vi "Auton Builder.vi"() -> ()   [LabVIEW 2019]
uses:
  Typedef/Robot Settings.ctl
  Typedef/Data Point.ctl
  Typedef/Robot Starting Position.ctl
  <vilib>/Rock Robotics/WPI/ThirdParty/WPILib Extensions/Trajectory/Typedef/Differential Drive Constraints.ctl
  <vilib>/Rock Robotics/WPI/ThirdParty/WPILib Extensions/Trajectory/Typedef/Differential Drive Constants.ctl
  Typedef/Landmark Definition.ctl
  Typedef/Sequence Command.ctl
  Typedef/Plate Arrangement.ctl
  <vilib>/Utility/miscctls.llb/LVRowAndColumnTypeDef.ctl
  <vilib>/Rock Robotics/WPI/ThirdParty/WPILib Extensions/Geometry/Typedef/Pose2d.ctl
  <vilib>/Rock Robotics/WPI/ThirdParty/WPILib Extensions/Geometry/Typedef/Translation2d.ctl
  <vilib>/Rock Robotics/WPI/ThirdParty/WPILib Extensions/Geometry/Typedef/Rotation2d.ctl
panel:
  in  "Start Position Names":T1=enum."Center"
  in  "Stop?":bool
  in  "Tab Control":enum32{"Builder", "Raw Sequence", "Settings"}(tab)
  in  "Landmarks":u16(ring) items=["Left Wall Start"]
  in  "Insert Landmark":bool
  in  "Alliance":bool
  out "Field Half":cluster{dbl[], dbl[]}[](graph)=[{[48.5, 82.0, 82.0, 48.5, 48.5], [176.25, 176.25, 147.75, 147.75, 176.25]}, {[68.0], [162.0]}, {[68.0], [162.0]}, {[81.13940299900052], [156.48469503745656]}, {[54.86059700099948], [167.51530496254344]}]
  in  "Start Position":T1=enum."Center"
  in  "Reverse Path":bool
  in  "Data Points":T2[](array[typedef])=[{"X"=68.0, "Y"=162.0, "Theta"=0.0, "Speed %"=0.0, "Disabled?"=FALSE}]
  in  "Open":bool
  in  "Save":bool
  in  "Reset":bool
  in  "Send to Robot":bool
  in  "Simulate":bool
  in  "Name":string
  in  "Cancel":bool
  out "Total Time Seconds":dbl
  in  "Lardmark List":T3[](array[typedef])=[{"X Red"=140.0, "Y Red"=305.0, "Theta Red"=0.0, "X Blue"=140.0, "Y Blue"=305.0, "Theta Blue"=0.0, "Name"="Left Wall Start"}]
  out "Location Names":string[](array[string])=["Top Center", "Center", "Bottom Center", "Top Railing"]
  in  "Locations":cluster{"X":dbl, "Y":dbl}[](array[cluster])=[{"X"=120.0, "Y"=266.0}, {"X"=120.0, "Y"=228.0}, {"X"=120.0, "Y"=187.0}, {"X"=120.0, "Y"=297.0}, {"X"=140.0, "Y"=305.0}]
  in  "Path Folder":path=path "C:/Users/RoboChargers/Documents/LabVIEW Data/Deep-Space-2019/Auton/Paths"
  in  "Robot Settings":T4={"Width"=0.6, "Length"=0.7, "Center of Rotation"=0.2} caption="Robot Settings w/ Bumpers"
  in  "Constants":T5={"ks"=0.162, "kv"=2.71, "ka"=0.468, "trackwidth"=0.67163}
  in  "Constraints":T6={"maxVoltage"=9.0, "maxVelocity"=3.0, "maxAccel"=1.5}
  # "LEFT"
  # "+Y"
  # "FAR"
  # "+X"
  # "NEAR"
  # "RIGHT"
  # "Counter Clockwise Positive\n+X = 0 degrees"
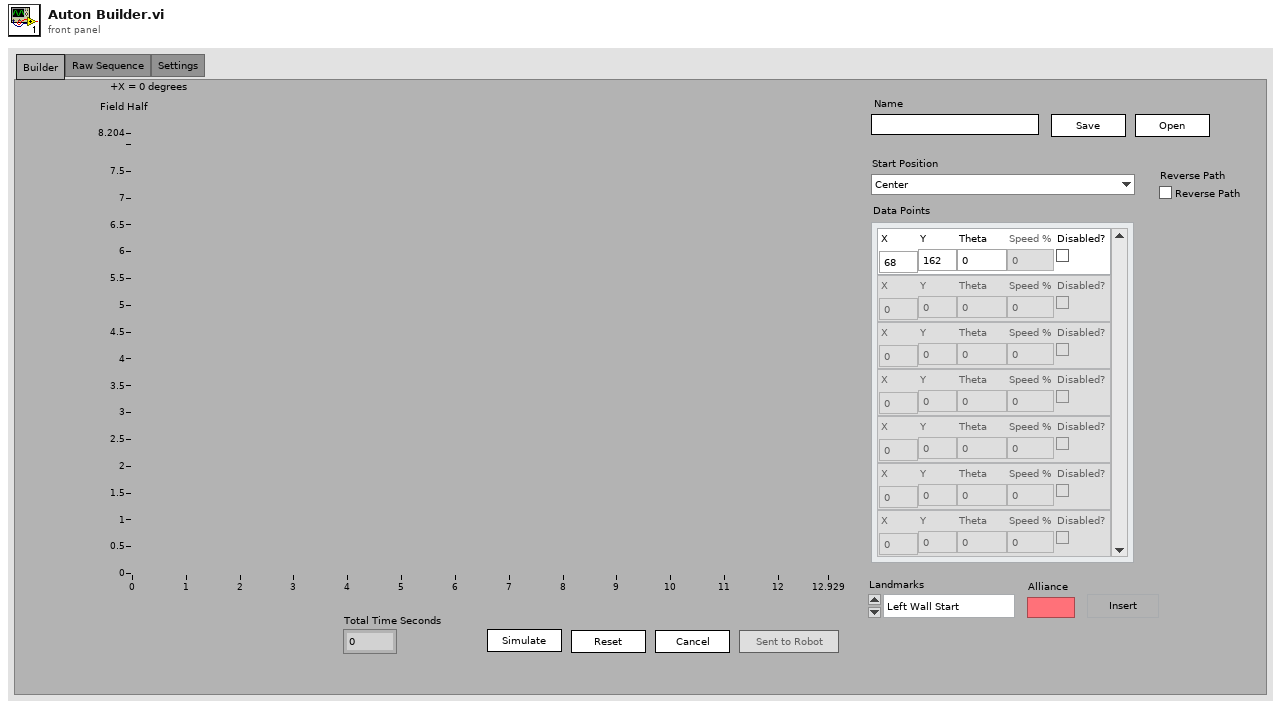
[diagram p1: front panel]
types:
  T1 = typedef "Robot Starting Position.ctl" = enum16{"Left Center", "Center", "Bottom Center", "Left Trench", "Left Wall"}
  T2 = typedef "Data Point.ctl" = cluster{"X":dbl, "Y":dbl, "Theta":dbl, "Speed %":dbl, "Disabled?":bool}
  T3 = typedef "Landmark Definition.ctl" = cluster{"X Red":dbl, "Y Red":dbl, "Theta Red":dbl, "X Blue":dbl, "Y Blue":dbl, "Theta Blue":dbl, "Name":string}
  T4 = typedef "Robot Settings.ctl" = cluster{"Width":dbl, "Length":dbl, "Center of Rotation":dbl}
  T5 = typedef "Differential Drive Constants.ctl" = cluster{"ks":dbl, "kv":dbl, "ka":dbl, "trackwidth":dbl}
  T6 = typedef "Differential Drive Constraints.ctl" = cluster{"maxVoltage":dbl, "maxVelocity":dbl, "maxAccel":dbl}
  T7 = typedef "Sequence Command.ctl" = cluster{"Sequence Name":string, "Plate Arrangement":T8, "Command Name":string, "Data":variant, "Sequence Number":u32}
  T8 = typedef "Plate Arrangement.ctl" = cluster{"LR*":bool, "LL*":bool, "RL*":bool, "RR*":bool}
  T9 = typedef "LVRowAndColumnTypeDef.ctl" = cluster{"Row":i32, "Column":i32}
  T10 = cluster{"Field Half":cluster{dbl[], dbl[]}[], "Current Command":T7, "Robot Position":cluster{"x":dbl, "y":dbl}, "Theta":dbl, "y position":dbl, "Active Cell":T9, "Robot Index":i32, "Sequence OK?":bool, "Start Position":cluster{"x":dbl, "y":dbl}, "Field Selection":string, "Simulation Index":i32, "Sim Robot Index":i32, "Active Path":path, "Load Index":i32, "Graph Index":i32, "Data Points Index":i32, "Data Points":T2[], "Path Index":i32, "Path L Index":i32, "Path R Index":i32}
  T11 = typedef "Pose2d.ctl" = cluster{"Translation2d":T12, "Rotation2d":T13}
  T12 = typedef "Translation2d.ctl" = cluster{"x":dbl, "y":dbl}
  T13 = typedef "Rotation2d.ctl" = cluster{"Theta":dbl}
  T14 = typedef "Trajectory State.ctl" = cluster{"t":dbl, "velocity":dbl, "acceleration":dbl, "pose":T11, "curvature":dbl}
  T15 = typedef "LVPoint32TypeDef.ctl" = cluster{"Horizontal":i32, "Vertical":i32}
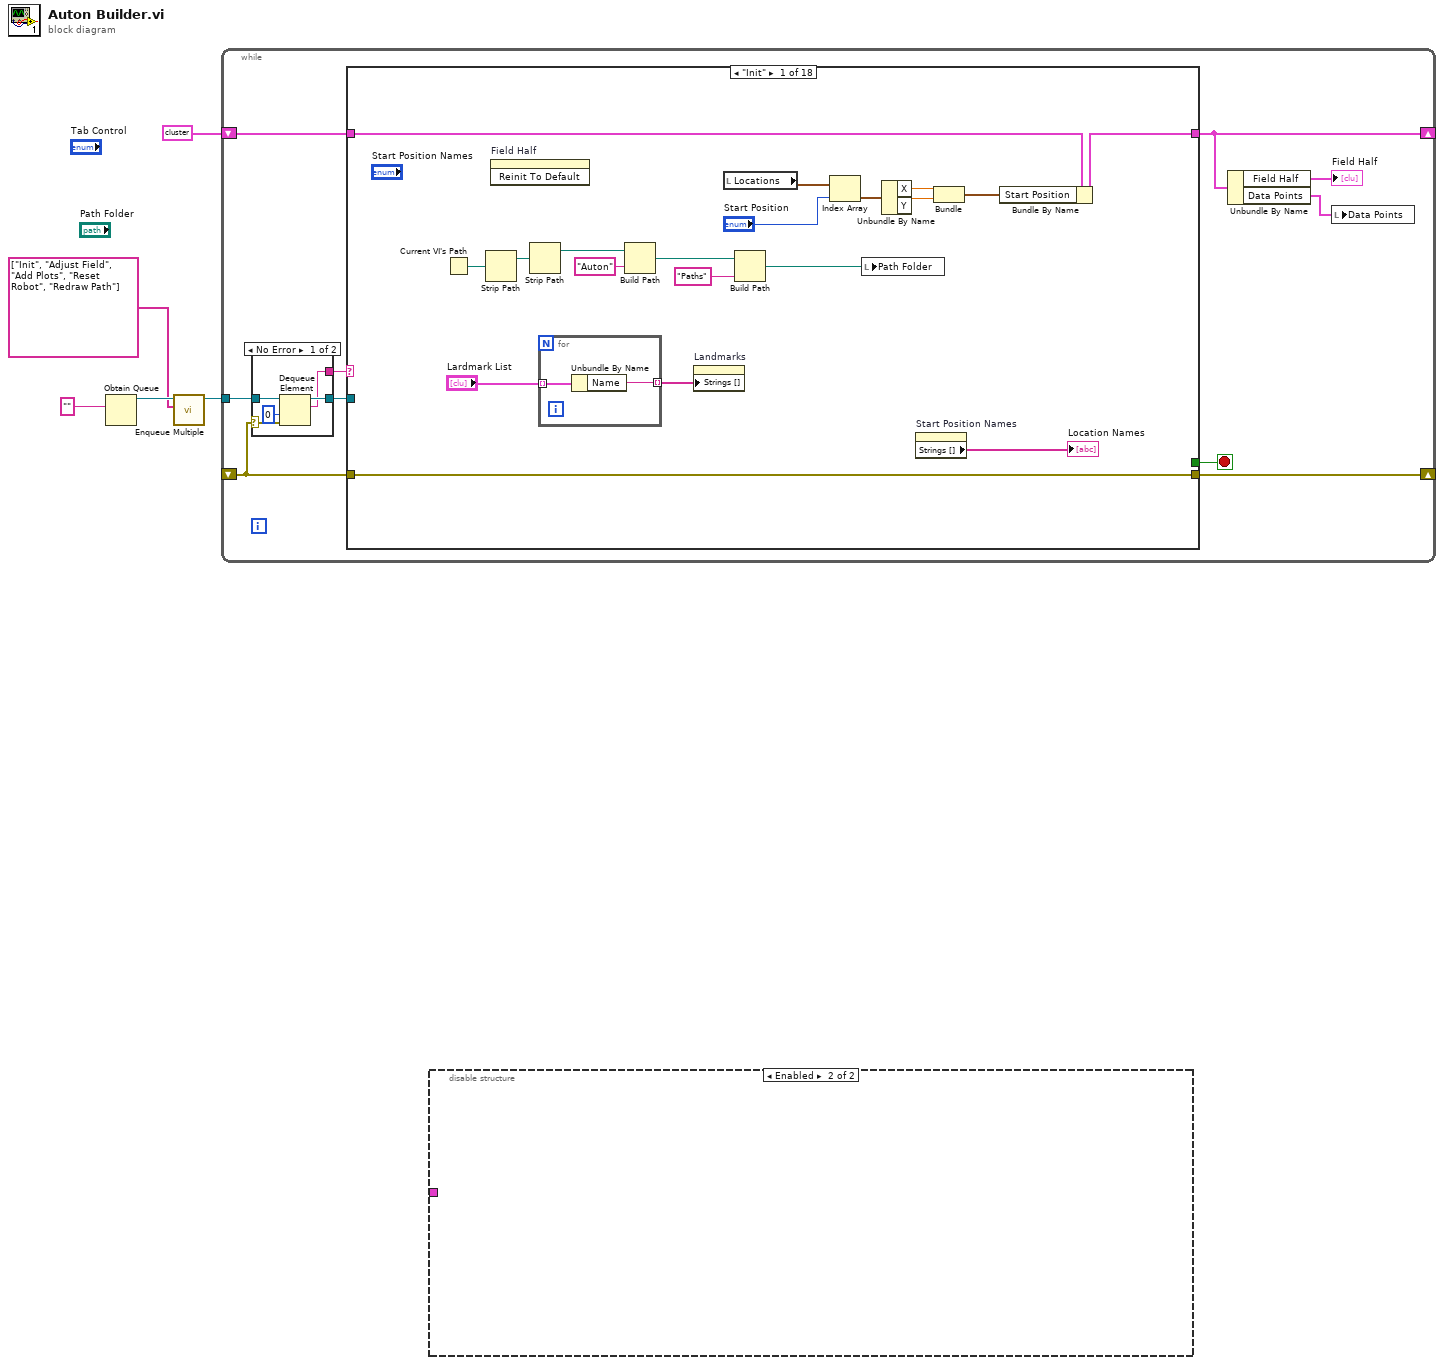
[diagram p0: block diagram]
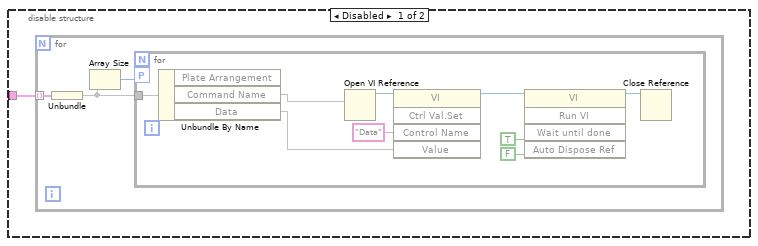
[diagram p2: hidden frame]
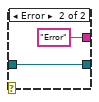
[diagram p3: hidden frame]
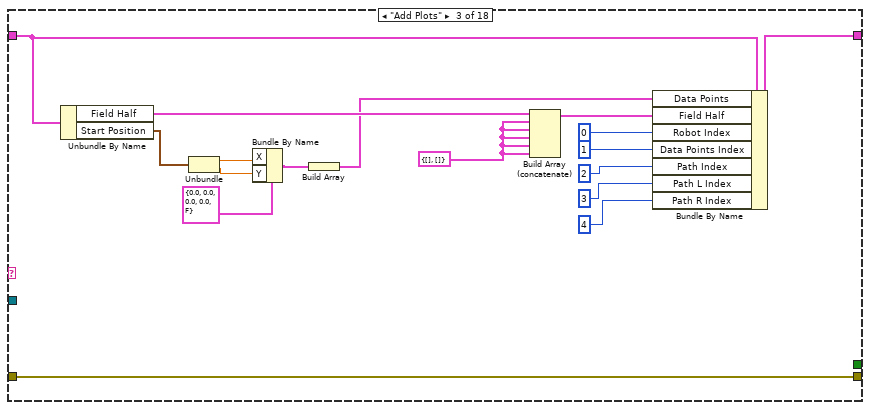
[diagram p5: hidden frame]
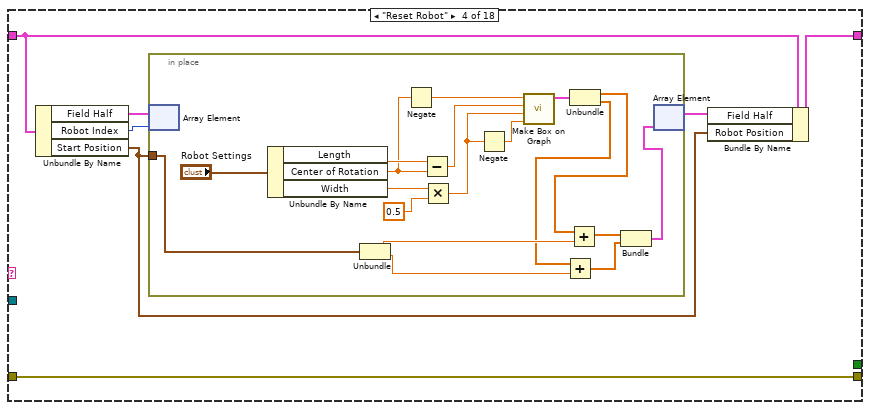
[diagram p6: hidden frame]
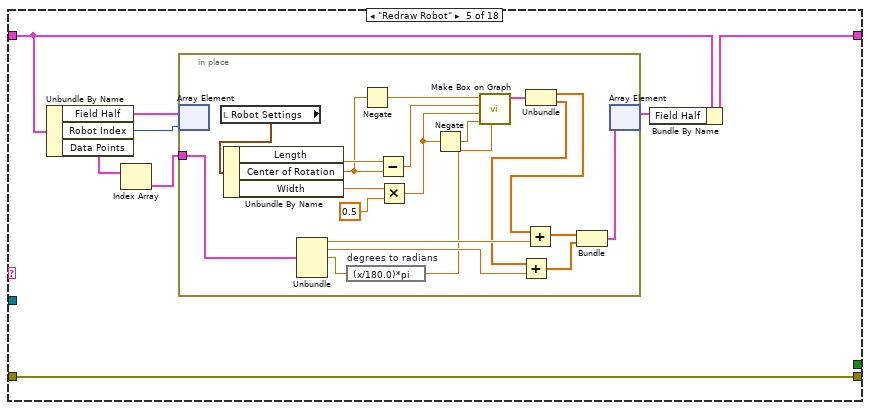
[diagram p7: hidden frame]
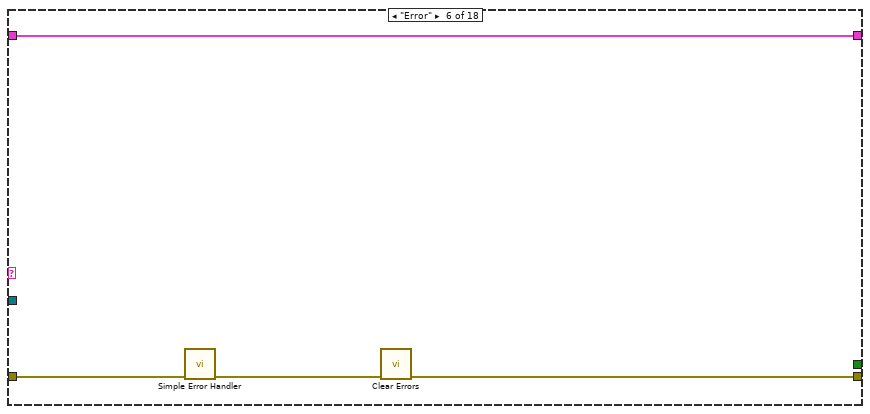
[diagram p8: hidden frame]
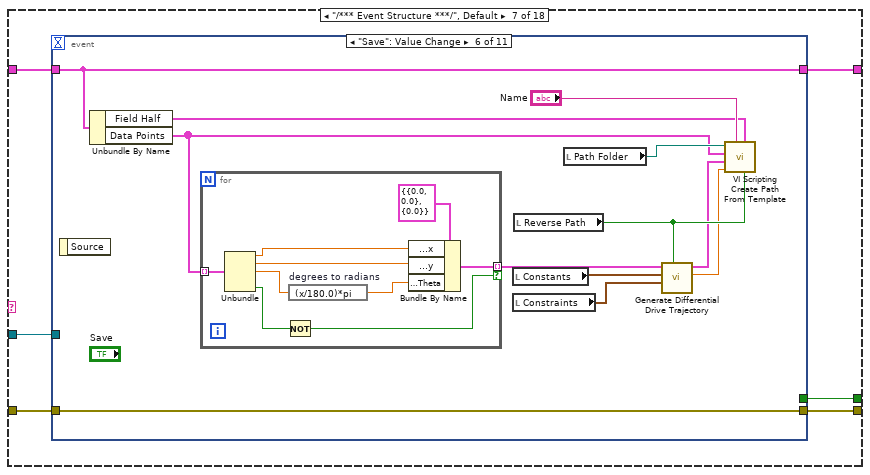
[diagram p9: hidden frame]
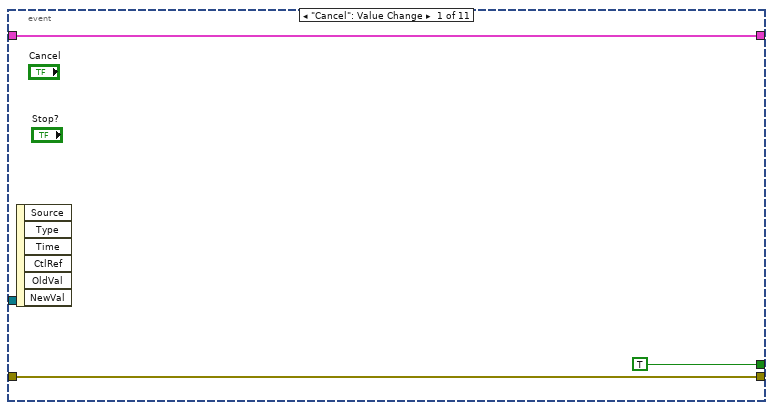
[diagram p10: hidden frame]
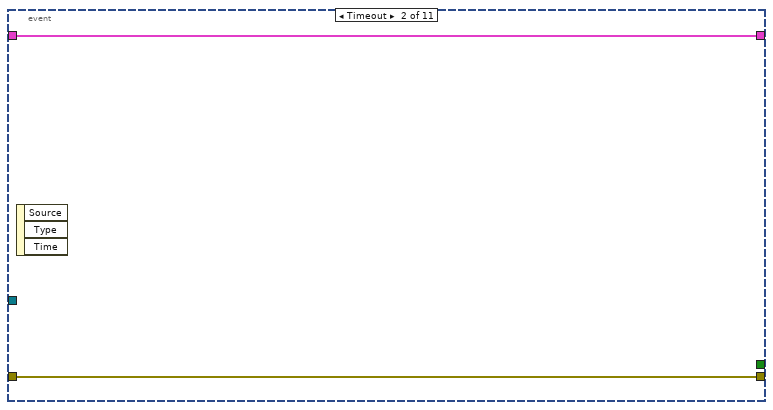
[diagram p11: hidden frame]
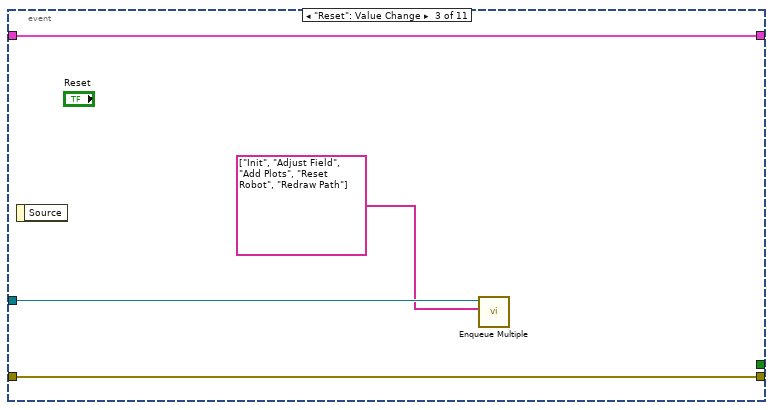
[diagram p12: hidden frame]
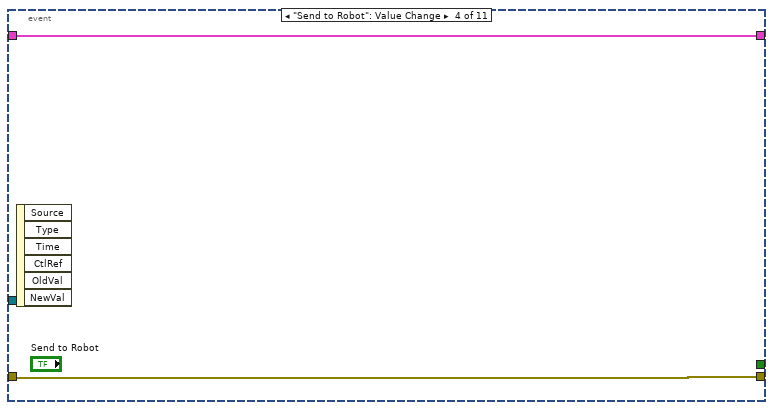
[diagram p13: hidden frame]
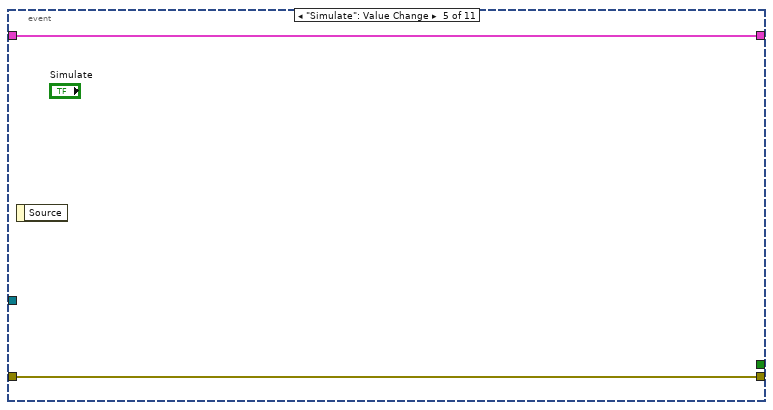
[diagram p14: hidden frame]
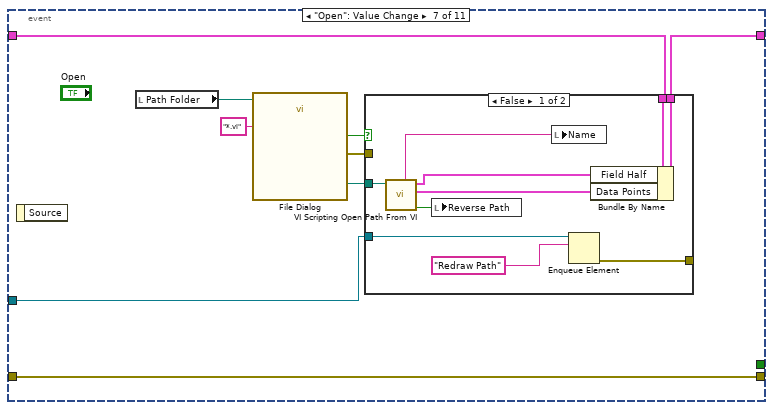
[diagram p15: hidden frame]
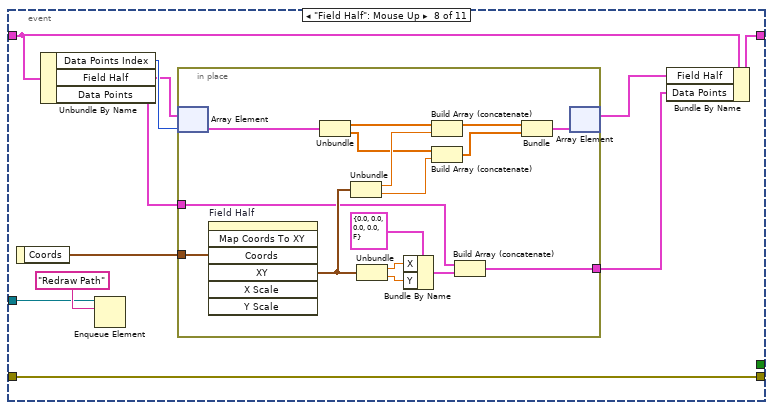
[diagram p17: hidden frame]
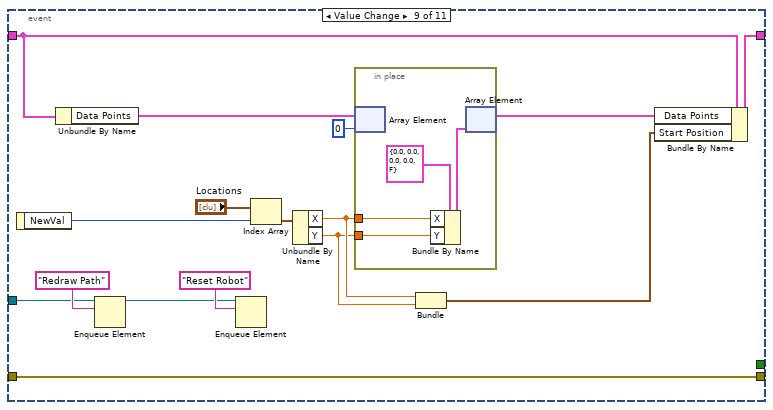
[diagram p18: hidden frame]
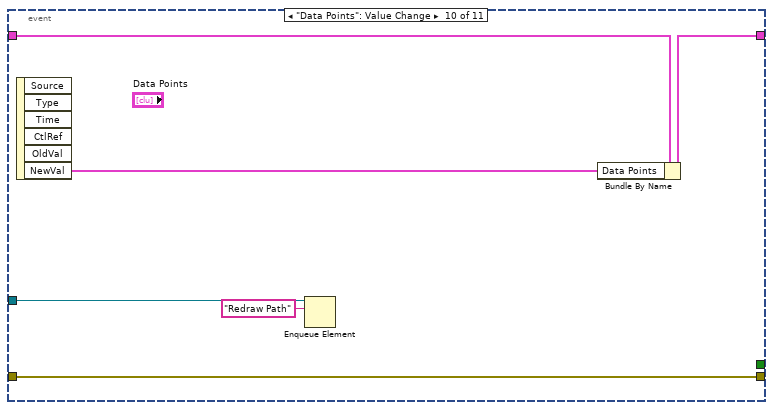
[diagram p19: hidden frame]
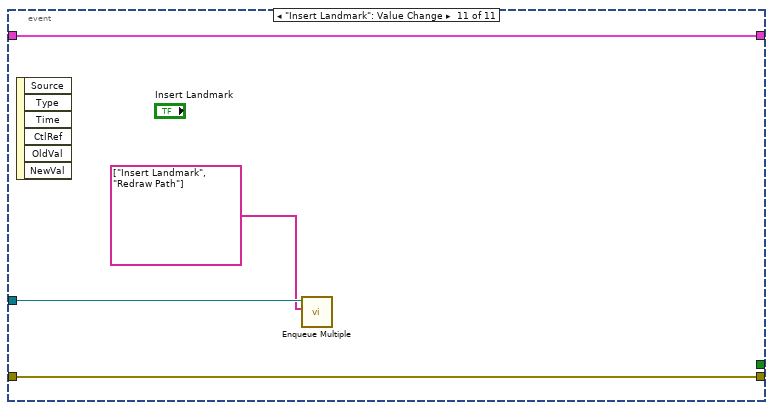
[diagram p20: hidden frame]
diagram:
  n1 = Obtain Queue(element data type="") -> (queue out=w4:refnum<queue>)  [unwired: 4 in, 2 out]
  n2 = call "Enqueue Multiple.vi"("Array"=string[] ["Init", "Adjust Field", "Add Plots", "Reset Robot", "Redraw Path"], "Queue in"=w4) -> ("Queue out"=w3:refnum<queue>)  [unwired: 8 in, 1 out]
  n3 = while {
    shift-right: [w9] -> _
    shift-left: T10 {"Field Half"=[], "Current Command"={"Sequence Name"="", "Plate Arrangement"={"LR*"=FALSE, "LL*"=FALSE, "RL*"=FALSE, "RR*"=FALSE}, "Command Name"="", "Data"=variant, "Sequence Number"=0}, "Robot Position"={"x"=0.0, "y"=0.0}, "Theta"=0.0, "y position"=0.0, "Active Cell"={"Row"=0, "Column"=0}, "Robot Index"=0, "Sequence OK?"=FALSE, "Start Position"={"x"=0.0, "y"=0.0}, "Field Selection"="", "Simulation Index"=0, "Sim Robot Index"=0, "Active Path"=path "", "Load Index"=0, "Graph Index"=0, "Data Points Index"=0, "Data Points"=[], "Path Index"=0, "Path L Index"=0, "Path R Index"=0} ("output cluster") -> [w15]
    shift-right: [w11] -> _
    shift-left: _ -> [w10]
    tunnel: w3 -> [w14]
    stop <- w7 stop-if-true
    n4 = case shown="No Error" w10 {
      selector: w10 -> [w18 _]
      tunnel: w14 -> [w20 w22]
      tunnel: [w19 w22] -> w13
      tunnel: [w17 "Error"] -> w12
      frame No Error {
        n5 = Dequeue Element(queue=w20, timeout in ms (-1)=0, error in (no error)=w18) -> (queue out=w19:refnum<queue>, element=w17:string)  [unwired: 2 out]
      }
      frame Error {
      }
    }
    n6 = case shown="\"Init\"" w12 {
      tunnel: [_ _ _ _ _ _ w125 _ _ _ _ _ _ _ _ _ _ _] -> w7
      tunnel: w15 -> [w41 w44 w60 w68 w94 w119 w124 w239 w251 w266 w278 w294 w336 w386 w401 w406 w408 w410]
      tunnel: [w40 w44 w62 w69 w95 w119 w123 w238 w244 w262 w277 w292 w334 w385 w401 w404 w408 w410] -> w9
      tunnel: w13 -> [_ _ _ _ _ _ w122 _ _ _ _ w285 w327 _ _ _ _ _]
      tunnel: [w39 w45 w58 w67 w93 w118 w120 w240 w242 w260 w279 w295 w337 w387 w400 w405 w407 w409] -> w11
      tunnel: w10 -> [w39 w45 w58 w67 w93 w117 w121 w240 w242 w260 w279 w295 w337 w387 w400 w405 w407 w409]
      frame "Init" {
        n7 = Current VI's Path() -> (path=w38:path)
        n8 = Strip Path(path=w38) -> (stripped path=w37:path)  [unwired: 1 out]
        n9 = invoke on="Field Half" class="XYGraph (strict)" method="Reinit To Default"() -> ()  [unwired: 3 in, 3 out]
        n10 = Strip Path(path=w37) -> (stripped path=w36:path)  [unwired: 1 out]
        n11 = for {
          tunnel: [w42] -> w23 mode=indexing
          tunnel: "Lardmark List" -> [w43] mode=indexing
          n12 = Unbundle By Name(w43) -> ("Name"=w42:string)
        }
        n13 = Build Path(base path=w36, name or relative path="Auton") -> (appended path=w34:path)
        n14 = property on="Landmarks" class="Ring (strict)"("Strings []"=w23) -> ()  [unwired: 2 in, 2 out]
        n15 = local read "Locations"() -> (w26:cluster{"X":dbl, "Y":dbl}[])
        n16 = Build Path(base path=w34, name or relative path="Paths") -> (appended path=w32:path)
        n17 = Index Array(array=w26, index="Start Position") -> (element=w30:cluster{"X":dbl, "Y":dbl})
        n18 = local write "Path Folder"(w32) -> ()
        n19 = Unbundle By Name(w30) -> ("X"=w29:dbl, "Y"=w28:dbl)
        n20 = property on="Start Position Names" class="Enum (strict)"() -> ("Strings []"=→"Location Names":string[])  [unwired: 2 in, 2 out]
        n21 = Bundle("X"=w29, "Y"=w28) -> (w27:cluster{"X":dbl, "Y":dbl})  [unwired: 1 in]
        n22 = Bundle By Name(cluster=w41, "Start Position"=w27) -> (w40:T10)
      }
      frame "Adjust Field" {
      }
      frame "Add Plots" {
        w51 = cluster{dbl[], dbl[]} {[], []} ("element")
        n23 = Unbundle By Name(w60) -> ("Field Half"=w59:cluster{dbl[], dbl[]}[], "Start Position"=w52:cluster{"x":dbl, "y":dbl})
        n24 = Unbundle(w52) -> ("x"=w49:dbl, "y"=w48:dbl)
        n25 = Bundle By Name(cluster=T2 {"X"=0.0, "Y"=0.0, "Theta"=0.0, "Speed %"=0.0, "Disabled?"=FALSE} ("Cluster"), "X"=w49, "Y"=w48) -> (w47:T2)
        n26 = Build Array(w47) -> (w46:T2[])
        n27 = Build Array (concatenate)(w59, w51, w51, w51, w51, w51) -> (w61:cluster{dbl[], dbl[]}[])
        n28 = Bundle By Name(cluster=w60, "Data Points"=w46, "Field Half"=w61, "Robot Index"=0, "Data Points Index"=1 ("Spline Index"), "Path Index"=2 ("Spline Index"), "Path L Index"=3 ("Spline Index"), "Path R Index"=4 ("Spline Index")) -> (w62:T10)
      }
      frame "Reset Robot" {
        n29 = Unbundle By Name(w68) -> ("Field Half"=w66:cluster{dbl[], dbl[]}[], "Robot Index"=w65:i32, "Start Position"=w63:cluster{"x":dbl, "y":dbl})
        n30 = in-place {
          in-place-border: w63 -> [w87]
          n31 = in-place-array #1(w66, w65) -> ()  [unwired: 1 out]
          n32 = Unbundle By Name("Robot Settings") -> ("Length"=w77:dbl, "Center of Rotation"=w76:dbl, "Width"=w81:dbl)
          n33 = Unbundle(w87) -> ("x"=w86:dbl, "y"=w85:dbl)
          n34 = Negate(x=w76) -> (-x=w78:dbl)
          n35 = Subtract(x=w77, y=w76) -> (x-y=w75:dbl)
          n36 = Multiply(x=w81, y=0.5 ("x")) -> (x*y=w80:dbl)
          n37 = Negate(x=w80) -> (-x=w79:dbl)
          n38 = call "Make Box on Graph.vi"("Y2"=w79, "Y1"=w80, "X2"=w75, "X1"=w78) -> ("Output Graph"=w73:cluster{dbl[], dbl[]})  [unwired: 7 in]
          n39 = Unbundle(w73) -> (w72:dbl[], w71:dbl[])
          n40 = Add(x=w71, y=w85) -> (x+y=w84:dbl[])
          n41 = Add(x=w72, y=w86) -> (x+y=w83:dbl[])
          n42 = Bundle(w83, w84) -> (w70:cluster{dbl[], dbl[]})  [unwired: 1 in]
          n43 = in-place-array #1(w70) -> (w64:cluster{dbl[], dbl[]}[])  [unwired: 1 out]
        }
        n44 = Bundle By Name(cluster=w68, "Field Half"=w64, "Robot Position"=w63) -> (w69:T10)
      }
      frame "Redraw Robot" {
        n45 = Unbundle By Name(w94) -> ("Field Half"=w92:cluster{dbl[], dbl[]}[], "Robot Index"=w91:i32, "Data Points"=w90:T2[])
        n46 = Index Array(array=w90) -> (element=w89:T2)  [unwired: 1 in]
        n47 = in-place {
          in-place-border: w89 -> [w115]
          n48 = in-place-array #2(w92, w91) -> ()  [unwired: 1 out]
          n49 = local read "Robot Settings"() -> (w99:T4)
          n50 = Unbundle By Name(w99) -> ("Length"=w106:dbl, "Center of Rotation"=w105:dbl, "Width"=w110:dbl)
          n51 = Unbundle(w115) -> ("X"=w114:dbl, "Y"=w113:dbl, "Theta"=w97:dbl)  [unwired: 2 out]
          n52 = expression code="(x/180.0)*pi" "degrees to radians"(w97) -> (w96:dbl)
          n53 = Negate(x=w105) -> (-x=w107:dbl)
          n54 = Subtract(x=w106, y=w105) -> (x-y=w104:dbl)
          n55 = Multiply(x=w110, y=0.5 ("x")) -> (x*y=w109:dbl)
          n56 = Negate(x=w109) -> (-x=w108:dbl)
          n57 = call "Make Box on Graph.vi"("Theta"=w96, "Y2"=w108, "Y1"=w109, "X2"=w104, "X1"=w107) -> ("Output Graph"=w102:cluster{dbl[], dbl[]})  [unwired: 6 in]
          n58 = Unbundle(w102) -> (w101:dbl[], w100:dbl[])
          n59 = Add(x=w100, y=w113) -> (x+y=w112:dbl[])
          n60 = Add(x=w101, y=w114) -> (x+y=w111:dbl[])
          n61 = Bundle(w111, w112) -> (w98:cluster{dbl[], dbl[]})  [unwired: 1 in]
          n62 = in-place-array #2(w98) -> (w88:cluster{dbl[], dbl[]}[])  [unwired: 1 out]
        }
        n63 = Bundle By Name(cluster=w94, "Field Half"=w88) -> (w95:T10)
      }
      frame "Error" {
        n64 = call <vilib>:"Simple Error Handler.vi"("error in (no error)"=w117) -> ("error out"=w116:errorcluster)  [unwired: 4 in, 4 out]
        n65 = call <vilib>:"Clear Errors.vi"("error in (no error)"=w116) -> ("error out"=w118:errorcluster)  [unwired: 5 in, 1 out]
      }
      frame "/*** Event Structure ***/", Default {
        n66 = event shown="[5] \"Save\": Value Change" {
          selector: _ -> [_ _ _ _ _ _ _ _ _ _ _]
          dyn-events: _ -> [_ _ _ _ _ _ _ _ _ _ _]
          timeout: _ -> [_ _ _ _ _ _ _ _ _ _ _]
          tunnel: [TRUE _ _ _ _ _ _ _ _ _ _] -> w125
          tunnel: w124 -> [w127 w130 w134 w136 w138 w150 w162 w186 w221 w231 w233]
          tunnel: [w127 w130 w134 w136 w138 w150 w161 w184 w220 w230 w233] -> w123
          tunnel: w122 -> [_ _ w133 _ _ _ w160 w180 w218 w228 w235]
          tunnel: w121 -> [w126 w129 w132 w135 w137 w148 w168 w190 w222 w232 w236]
          tunnel: [w126 w129 w132 w135 w137 w148 w168 w190 w222 w232 w236] -> w120
          event "Cancel": Value Change {
            n67 = event-data() -> ()  [unwired: 1 in, 6 out]
          }
          event Timeout {
            n68 = event-data() -> ()  [unwired: 1 in, 3 out]
          }
          event "Reset": Value Change {
            n69 = event-data() -> ()  [unwired: 1 in, 1 out]
            n70 = call "Enqueue Multiple.vi"("Array"=string[] ["Init", "Adjust Field", "Add Plots", "Reset Robot", "Redraw Path"], "Queue in"=w133) -> ()  [unwired: 8 in, 2 out]
          }
          event "Send to Robot": Value Change {
            n71 = event-data() -> ()  [unwired: 1 in, 6 out]
          }
          event "Simulate": Value Change {
            n72 = event-data() -> ()  [unwired: 1 in, 1 out]
          }
          event "Save": Value Change {
            n73 = event-data() -> ()  [unwired: 1 in, 1 out]
            n74 = Unbundle By Name(w150) -> ("Field Half"=w146:cluster{dbl[], dbl[]}[], "Data Points"=w142:T2[])
            n75 = for {
              tunnel: w142 -> [w159] mode=indexing
              tunnel: [w157] -> w145 mode=indexing if=w155
              n76 = Unbundle(w159) -> ("X"=w151:dbl, "Y"=w152:dbl, "Theta"=w153:dbl, "Disabled?"=w156:bool)  [unwired: 1 out]
              n77 = Not(x=w156) -> (.not. x?=w155:bool)
              n78 = expression code="(x/180.0)*pi" "degrees to radians"(w153) -> (w154:dbl)
              n79 = Bundle By Name(cluster=T11 {"Translation2d"={"x"=0.0, "y"=0.0}, "Rotation2d"={"Theta"=0.0}} ("pose"), "Translation2d.x"=w151, "Translation2d.y"=w152, "Rotation2d.Theta"=w154) -> (w157:T11)
            }
            n80 = local read "Constants"() -> (w143:T5)
            n81 = local read "Constraints"() -> (w144:T6)
            n82 = local read "Reverse Path"() -> (w141:bool)
            n83 = local read "Path Folder"() -> (w147:path)
            n84 = call <vilib>:"Generate Differential Drive Trajectory.vi"("Reverse?"=w141, "Constraints"=w144, "Constants"=w143, "Waypoints"=w145) -> ("Total Time Seconds"=w139:dbl, "states"=w140:T14[])  [unwired: 5 in, 1 out]
            n85 = call "VI Scripting Create Path From Template.vi"("Reverse Path?"=w141, "Graph"=w146, "Name"="Name", "Total Time (s)"=w139, "Trajectory"=w140, "Data Points"=w142, "base path"=w147) -> ()  [unwired: 5 in]
          }
          event "Open": Value Change {
            n86 = event-data() -> ()  [unwired: 1 in, 1 out]
            n87 = local read "Path Folder"() -> (w166:path)
            n88 = call "File Dialog"("start path"=w166, "pattern (all files)"="*.vi") -> ("selected path"=w167:path, "cancelled"=w165:bool, "error out"=w164:errorcluster)  [unwired: 10 in, 1 out]
            n89 = case shown="False" w165 {
              tunnel: w167 -> [w178 _]
              tunnel: w162 -> [w177 w179]
              tunnel: [w175 w179] -> w161
              tunnel: w160 -> [w172 _]
              tunnel: w164 -> [_ _]
              tunnel: [w169 _] -> _
              frame False {
                n90 = call "VI Scripting Open Path From VI.vi"("Path"=w178) -> ("Reverse Path?"=w176:bool, "Data Points"=w173:T2[], "Graph"=w174:cluster{dbl[], dbl[]}[], "Name"=w170:string)  [unwired: 6 in, 1 out]
                n91 = local write "Reverse Path"(w176) -> ()
                n92 = local write "Name"(w170) -> ()
                n93 = Enqueue Element(queue=w172, element="Redraw Path") -> (error out=w169:errorcluster)  [unwired: 2 in, 2 out]
                n94 = Bundle By Name(cluster=w177, "Field Half"=w174, "Data Points"=w173) -> (w175:T10)
              }
              frame True {
              }
            }
          }
          event "Field Half": Mouse Up {
            n95 = event-data() -> ("Coords"=w189:T15)  [unwired: 1 in]
            n96 = Unbundle By Name(w186) -> ("Data Points Index"=w188:i32, "Field Half"=w187:cluster{dbl[], dbl[]}[], "Data Points"=w182:T2[])
            n97 = Enqueue Element(queue=w180, element="Redraw Path") -> ()  [unwired: 2 in, 3 out]
            n98 = in-place {
              in-place-border: w189 -> [w198]
              in-place-border: [w192] -> w183
              in-place-border: w182 -> [w191]
              n99 = in-place-array #3(w187, w188) -> (w206:cluster{dbl[], dbl[]})
              n100 = invoke on="Field Half" class="XYGraph (strict)" method="Map Coords To XY"("Coords"=w198) -> ("XY"=w196:cluster{"X":dbl, "Y":dbl})  [unwired: 6 in, 6 out]
              n101 = Unbundle(w206) -> (w204:dbl[], w203:dbl[])
              n102 = Unbundle(w196) -> ("X"=w205:dbl, "Y"=w202:dbl)
              n103 = Unbundle(w196) -> ("X"=w195:dbl, "Y"=w194:dbl)
              n104 = Bundle By Name(cluster=T2 {"X"=0.0, "Y"=0.0, "Theta"=0.0, "Speed %"=0.0, "Disabled?"=FALSE} ("Cluster"), "X"=w195, "Y"=w194) -> (w197:T2)
              n105 = Build Array (concatenate)(w204, w205) -> (w201:dbl[])
              n106 = Build Array (concatenate)(w203, w202) -> (w200:dbl[])
              n107 = Build Array (concatenate)(w191, w197) -> (w192:T2[])
              n108 = Bundle(w201, w200) -> (w199:cluster{dbl[], dbl[]})  [unwired: 1 in]
              n109 = in-place-array #3(w199) -> (w185:cluster{dbl[], dbl[]}[])  [unwired: 1 out]
            }
            n110 = Bundle By Name(cluster=w186, "Field Half"=w185, "Data Points"=w183) -> (w184:T10)
          }
          event Value Change {
            n111 = event-data() -> ("NewVal"=w212:T1)  [unwired: 1 in]
            n112 = Unbundle By Name(w221) -> ("Data Points"=w216:T2[])
            n113 = Enqueue Element(queue=w218, element="Redraw Path") -> (queue out=w210:refnum<queue>)  [unwired: 2 in, 2 out]
            n114 = Enqueue Element(queue=w210, element="Reset Robot") -> ()  [unwired: 2 in, 3 out]
            n115 = Index Array(array="Locations", index=w212) -> (element=w213:cluster{"X":dbl, "Y":dbl})
            n116 = Unbundle By Name(w213) -> ("X"=w209:dbl, "Y"=w208:dbl)
            n117 = in-place {
              in-place-border: w209 -> [w224]
              in-place-border: w208 -> [w223]
              n118 = in-place-array #4(w216, 0) -> ()  [unwired: 1 out]
              n119 = Bundle By Name(cluster=T2 {"X"=0.0, "Y"=0.0, "Theta"=0.0, "Speed %"=0.0, "Disabled?"=FALSE} ("element"), "X"=w224, "Y"=w223) -> (w226:T2)
              n120 = in-place-array #4(w226) -> (w217:T2[])  [unwired: 1 out]
            }
            n121 = Bundle("X"=w209, "Y"=w208) -> (w207:cluster{"X":dbl, "Y":dbl})  [unwired: 1 in]
            n122 = Bundle By Name(cluster=w221, "Data Points"=w217, "Start Position"=w207) -> (w220:T10)
          }
          event "Data Points": Value Change {
            n123 = event-data() -> ("NewVal"=w229:T2[])  [unwired: 1 in, 5 out]
            n124 = Enqueue Element(queue=w228, element="Redraw Path") -> ()  [unwired: 2 in, 3 out]
            n125 = Bundle By Name(cluster=w231, "Data Points"=w229) -> (w230:T10)
          }
          event "Insert Landmark": Value Change {
            n126 = event-data() -> ()  [unwired: 1 in, 6 out]
            n127 = call "Enqueue Multiple.vi"("Array"=string[] ["Insert Landmark", "Redraw Path"], "Queue in"=w235) -> ()  [unwired: 8 in, 2 out]
          }
        }
      }
      frame "Check Auton Sequence" {
        n128 = Bundle By Name(cluster=w239, "Sequence OK?"=FALSE) -> (w238:T10)
      }
      frame "Handle Graph Delete" {
        n129 = Unbundle By Name(w251) -> ("Field Half"=w245:cluster{dbl[], dbl[]}[], "Current Command"=w250:T7)
        n130 = Unbundle By Name(w250) -> ("Data"=w249:variant)
        n131 = Get Variant Attribute(Variant=w249, name="_graphIndex", default value (empty Variant)=0) -> (found=w241:bool, value=w247:i32)  [unwired: 1 in, 2 out]
        n132 = case shown="True" w241 {
          tunnel: w247 -> [_ w255]
          tunnel: w245 -> [w252 w254]
          tunnel: [w252 w253] -> w243
          frame False {
          }
          frame True {
            n133 = in-place {
              n134 = in-place-array #5(w254, w255) -> ()  [unwired: 1 out]
              n135 = in-place-array #5(cluster{dbl[], dbl[]} {[], []} ("element")) -> (w253:cluster{dbl[], dbl[]}[])  [unwired: 1 out]
            }
          }
        }
        n136 = Bundle By Name(cluster=w251, "Field Half"=w243) -> (w244:T10)
      }
      frame "Add Robot Plot" {
        n137 = Unbundle By Name(w266) -> ("Field Half"=w259:cluster{dbl[], dbl[]}[], "Current Command.Data"=w265:variant)
        n138 = Index Array(array=w259) -> (element=w257:cluster{dbl[], dbl[]})  [unwired: 1 in]
        n139 = Get Variant Attribute(Variant=w265, name="_graphPlot") -> (found=w263:bool, value=w258:variant)  [unwired: 2 in, 2 out]
        n140 = case shown="True" w263 {
          tunnel: [w267 w272] -> w261
          tunnel: w259 -> [w267 w271]
          tunnel: w258 -> [_ w270]
          tunnel: w257 -> [_ w269]
          frame False {
          }
          frame True {
            n141 = Variant To Data(type=w269, Variant=w270) -> (data=w268:cluster{dbl[], dbl[]})  [unwired: 1 in, 1 out]
            n142 = Build Array (concatenate)(w271, w268) -> (w272:cluster{dbl[], dbl[]}[])
          }
        }
        n143 = Bundle By Name(cluster=w266, "Field Half"=w261) -> (w262:T10)
      }
      frame "Update Graph Index" {
        n144 = Unbundle By Name(w278) -> ("Field Half"=w276:cluster{dbl[], dbl[]}[], "Graph Index"=w275:i32, "Current Command.Data"=w274:variant)
        n145 = in-place {
          in-place-border: w274 -> [w282]
          n146 = in-place-array #6(w276, w275) -> ()  [unwired: 1 out]
          n147 = Get Variant Attribute(Variant=w282, name="_graphPlot", default value (empty Variant)=cluster{dbl[], dbl[]} {[], []} ("value")) -> (value=w280:cluster{dbl[], dbl[]})  [unwired: 1 in, 3 out]
          n148 = in-place-array #6(w280) -> (w273:cluster{dbl[], dbl[]}[])  [unwired: 1 out]
        }
        n149 = Bundle By Name(cluster=w278, "Field Half"=w273) -> (w277:T10)
      }
      frame "Redraw Path" {
        n150 = Unbundle By Name(w294) -> ("Data Points"=w290:T2[], "Field Half"=w293:cluster{dbl[], dbl[]}[], "Data Points Index"=w286:i32, "Path Index"=w287:i32, "Path L Index"=w288:i32, "Path R Index"=w289:i32)
        n151 = Enqueue Element(queue=w285, element="Redraw Robot") -> ()  [unwired: 2 in, 3 out]
        n152 = in-place {
          in-place-border: w290 -> [w310]
          n153 = in-place-array #7(w293, w286, w287, w288, w289) -> ()  [unwired: 4 out]
          n154 = for {
            tunnel: w310 -> [w325] mode=indexing
            tunnel: [w323] -> w306 mode=indexing
            tunnel: [w322] -> w305 mode=indexing
            tunnel: [w321] -> w301 mode=indexing if=w319
            n155 = Unbundle(w325) -> ("X"=w323:dbl, "Y"=w322:dbl, "Theta"=w318:dbl, "Disabled?"=w320:bool)  [unwired: 1 out]
            n156 = expression code="(x/180.0)*pi" ("degrees to radians")(w318) -> (w317:dbl)
            n157 = Not(x=w320) -> (.not. x?=w319:bool)
            n158 = Bundle By Name(cluster=T11 {"Translation2d"={"x"=0.0, "y"=0.0}, "Rotation2d"={"Theta"=0.0}} ("pose"), "Translation2d.x"=w323, "Translation2d.y"=w322, "Rotation2d.Theta"=w317) -> (w321:T11)
          }
          n159 = local read "Robot Settings"() -> (w303:T4)
          n160 = Unbundle By Name(w303) -> ("Width"=w302:dbl)
          n161 = call <vilib>:"Generate Differential Drive Trajectory.vi"("Reverse?"="Reverse Path", "Constraints"="Constraints", "Constants"="Constants", "Waypoints"=w301) -> ("Total Time Seconds"=→"Total Time Seconds":dbl, "states"=w297:T14[])  [unwired: 5 in, 1 out]
          n162 = for {
            tunnel: [w314] -> w312 mode=indexing
            tunnel: [w315] -> w313 mode=indexing
            tunnel: w297 -> [w316] mode=indexing
            n163 = Unbundle By Name(w316) -> ("pose.Translation2d.x"=w314:dbl, "pose.Translation2d.y"=w315:dbl)
          }
          n164 = Bundle(w306, w305) -> (w304:cluster{dbl[], dbl[]})  [unwired: 1 in]
          n165 = Bundle(w312, w313) -> (w307:cluster{dbl[], dbl[]})  [unwired: 1 in]
          n166 = call "Path to Wheel Path.vi"("Wheelbase (in)"=w302, "waypoints"=w307) -> ("out"=w311:cluster{dbl[], dbl[]}[])  [unwired: 9 in]
          n167 = Index Array(array=w311) -> (element #1=w308:cluster{dbl[], dbl[]}, element #2=w309:cluster{dbl[], dbl[]})  [unwired: 2 in]
          n168 = in-place-array #7(w304, w307, w308, w309) -> (w291:cluster{dbl[], dbl[]}[])  [unwired: 4 out]
        }
        n169 = Bundle By Name(cluster=w294, "Field Half"=w291) -> (w292:T10)
      }
      frame "Redraw Path - Old Method" {
        n170 = Unbundle By Name(w336) -> ("Data Points"=w332:T2[], "Field Half"=w335:cluster{dbl[], dbl[]}[], "Data Points Index"=w328:i32, "Path Index"=w329:i32, "Path L Index"=w330:i32, "Path R Index"=w331:i32)
        n171 = Enqueue Element(queue=w327, element="Redraw Robot") -> ()  [unwired: 2 in, 3 out]
        n172 = in-place {
          in-place-border: w332 -> [w346]
          n173 = in-place-array #8(w335, w328, w329, w330, w331) -> ()  [unwired: 4 out]
          n174 = for {
            tunnel: [w363] -> w351 mode=indexing
            tunnel: w346 -> [w362] mode=indexing
            tunnel: [w361] -> w342 mode=indexing
            tunnel: [w360] -> w341 mode=indexing
            n175 = Unbundle(w362) -> ("X"=w361:dbl, "Y"=w360:dbl)  [unwired: 3 out]
            n176 = Bundle("X"=w361, "Y"=w360) -> (w363:cluster{"X":dbl, "Y":dbl})  [unwired: 1 in]
          }
          n177 = local read "Robot Settings"() -> (w339:T4)
          n178 = call "Path Inject Points.vi"("Distance"=1.0, "Path"=w351) -> ("Path out"=w356:cluster{dbl, dbl}[])  [unwired: 9 in]
          n179 = Bundle(w342, w341) -> (w340:cluster{dbl[], dbl[]})  [unwired: 1 in]
          n180 = Unbundle By Name(w339) -> ("Width"=w338:dbl)
          n181 = call "Path Smoother.vi"("tolerance"=0.001, "B"=0.95, "A"=0.05, "Path"=w356) -> ("SmoothPath"=w350:cluster{dbl, dbl}[])  [unwired: 7 in]
          n182 = for {
            tunnel: w350 -> [w359] mode=indexing
            tunnel: [w358] -> w348 mode=indexing
            tunnel: [w357] -> w349 mode=indexing
            n183 = Unbundle(w359) -> (w358:dbl, w357:dbl)
          }
          n184 = Bundle(w348, w349) -> (w343:cluster{dbl[], dbl[]})  [unwired: 1 in]
          n185 = call "Path to Wheel Path.vi"("Wheelbase (in)"=w338, "waypoints"=w343) -> ("out"=w347:cluster{dbl[], dbl[]}[])  [unwired: 9 in]
          n186 = Index Array(array=w347) -> (element #1=w344:cluster{dbl[], dbl[]}, element #2=w345:cluster{dbl[], dbl[]})  [unwired: 2 in]
          n187 = in-place-array #8(w340, w343, w344, w345) -> (w333:cluster{dbl[], dbl[]}[])  [unwired: 4 out]
        }
        n188 = Bundle By Name(cluster=w336, "Field Half"=w333) -> (w334:T10)
      }
      frame "Insert Landmark" {
        # "Don't insert a \nduplicate"
        n189 = local read "Lardmark List"() -> (w384:T3[])
        n190 = Unbundle By Name(w386) -> ("Data Points"=w381:T2[])
        n191 = Index Array(array=w384, index="Landmarks") -> (element=w382:T3)
        n192 = Array Size(array=w381) -> (size(s)=w377:i32)
        n193 = case shown="False" "Alliance" {
          tunnel: w382 -> [w391 w395]
          tunnel: [w390 w394] -> w368
          tunnel: [w389 w393] -> w369
          tunnel: [w388 w392] -> w370
          frame True {
            # "Blue"
            n194 = Unbundle By Name(w391) -> ("X Blue"=w388:dbl, "Y Blue"=w389:dbl, "Theta Blue"=w390:dbl)
          }
          frame False {
            # "Red"
            n195 = Unbundle By Name(w395) -> ("X Red"=w392:dbl, "Y Red"=w393:dbl, "Theta Red"=w394:dbl)
          }
        }
        n196 = Decrement(x=w377) -> (x-1=w376:i32)
        n197 = Index Array(array=w381, index=w376) -> (element=w375:T2)
        n198 = Unbundle By Name(w375) -> ("X"=w373:dbl, "Y"=w372:dbl, "Theta"=w371:dbl)
        n199 = Equal?(x=w373, y=w370) -> (x = y?=w365:bool)
        n200 = Equal?(x=w372, y=w369) -> (x = y?=w366:bool)
        n201 = Equal?(x=w371, y=w368) -> (x = y?=w367:bool)
        n202 = Bundle By Name(cluster=T2 {"X"=0.0, "Y"=0.0, "Theta"=0.0, "Speed %"=0.0, "Disabled?"=FALSE} ("element"), "X"=w370, "Y"=w369, "Theta"=w368) -> (w378:T2)
        n203 = Compound Arithmetic op=AND(w365, w366, w367) -> (w364:bool)
        n204 = case shown="False" w364 {
          tunnel: w381 -> [w398 w399]
          tunnel: [w397 w399] -> w380
          tunnel: w378 -> [w396 _]
          frame False {
            n205 = Build Array (concatenate)(w398, w396) -> (w397:T2[])
          }
          frame True {
          }
        }
        n206 = Bundle By Name(cluster=w386, "Data Points"=w380) -> (w385:T10)
      }
      frame "/**** Simulation Functions ****/" {
      }
      frame "Simulation Init" {
        n207 = Bundle By Name(cluster=w406, "Simulation Index"=0, "Sim Robot Index"=0) -> (w404:T10)
      }
      frame "Select Field String" {
      }
      frame "/**** File Operations ****/" {
      }
    }
    n208 = Unbundle By Name(w9) -> ("Field Half"=→"Field Half":cluster{dbl[], dbl[]}[], "Data Points"=w6:T2[])
    n209 = local write "Data Points"(w6) -> ()
  }
  n210 = disable-structure shown="Enabled" {
    disable-tunnel: _ -> [w411 _]
    frame Disabled {
      n211 = for {
        tunnel: w411 -> [w414] mode=indexing
        n212 = Unbundle(w414) -> ("Sequence Array"=w412)
        n213 = Array Size(array=w412) -> (size(s)=w413:i32)
        n214 = for {
          tunnel: w412 -> [w423]
          workers-P: w413 -> [_]
          n215 = Unbundle By Name(w423) -> ("Command Name"=w419, "Data"=w421)  [unwired: 1 out]
          n216 = Open VI Reference(vi path=w419) -> (vi reference=w422:refnum<vi>)  [unwired: 5 in, 1 out]
          n217 = invoke class="VI" method="Ctrl Val.Set"(reference=w422, "Control Name"="Data", "Value"=w421) -> (reference out=w418:refnum<vi>)  [unwired: 2 in, 4 out]
          n218 = invoke class="VI" method="Run VI"(reference=w418, "Wait until done"=TRUE ("Wait Until Done"), "Auto Dispose Ref"=FALSE ("Auto Dispose Reference")) -> (reference out=w417:refnum<vi>)  [unwired: 2 in, 4 out]
          n219 = Close Reference(reference=w417) -> ()  [unwired: 1 in, 1 out]
        }
      }
    }
    frame Enabled {
    }
  }
